vi "Threshold Windows Host.vi"() -> ()   [LabVIEW 2010]
uses:
  <vilib>/userDefined/High Color/nirio_resource_hc.ctl
  <vilib>/rvi/interface/nirviOpenFPGA/nirviOpenFPGA.xnode
  Threshold FPGA.vi
  <vilib>/rvi/interface/nirviOpenFPGA/nirviOpenFPGA.ctl
  <vilib>/rvi/interface/nirviOpenFPGA/nirviopenstate.ctl
  <vilib>/picture/picture.llb/imagedata.ctl
  <vilib>/rvi/interface/common/nirviIntfCommonState.ctl
  <vilib>/rvi/interface/common/nirviIntfModes.ctl
  Program Files/National Instruments/LabVIEW 2010/resource/RVI/emulation/niLvFpgaEmulationMode.ctl
  <vilib>/eio/XNode/Errors/EIOXNodeErrorStruct.ctl
  <vilib>/eio/XNode/Errors/EIOXNodeInternalErrorTypes.ctl
  <vilib>/eio/XNode/Errors/EIOXNodeUserErrorTypes.ctl
  <vilib>/XNodeSupport/XNodeRect32.ctl
  <vilib>/XNodeSupport/XNodeInt.ctl
  <vilib>/XNodeSupport/XNodeTerms.ctl
  <vilib>/XNodeSupport/XNodeTerm.ctl
  <vilib>/XNodeSupport/XNodeString.ctl
  <vilib>/XNodeSupport/XNodeVariant.ctl
  <vilib>/XNodeSupport/XNodeBool.ctl
  <vilib>/rvi/interface/nirviReadWriteControl/nirviReadWriteControl.xnode
  <vilib>/rvi/interface/nirviCloseFPGA/nirviCloseFPGA.xnode
  <vilib>/rvi/interface/RandomDataEmulation/nirviRandomDataOpen.vi
  <vilib>/rvi/interface/RandomDataEmulation/nirviRandomDataClose.vi
  <vilib>/XNodeSupport/NI_XNodeSupport.lvlib
panel:
  in  "Threshold (Volts)":dbl
  out "AI0 (Volts)":dbl
  in  "Stop Host":bool
  out "Threshold Exceeded":bool
  in  "Monitoring Loop Period (ms)":u32
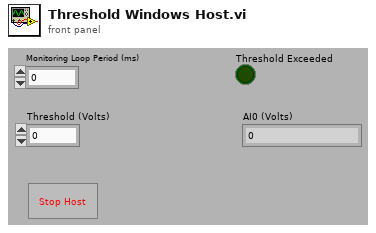
[diagram p1: front panel]
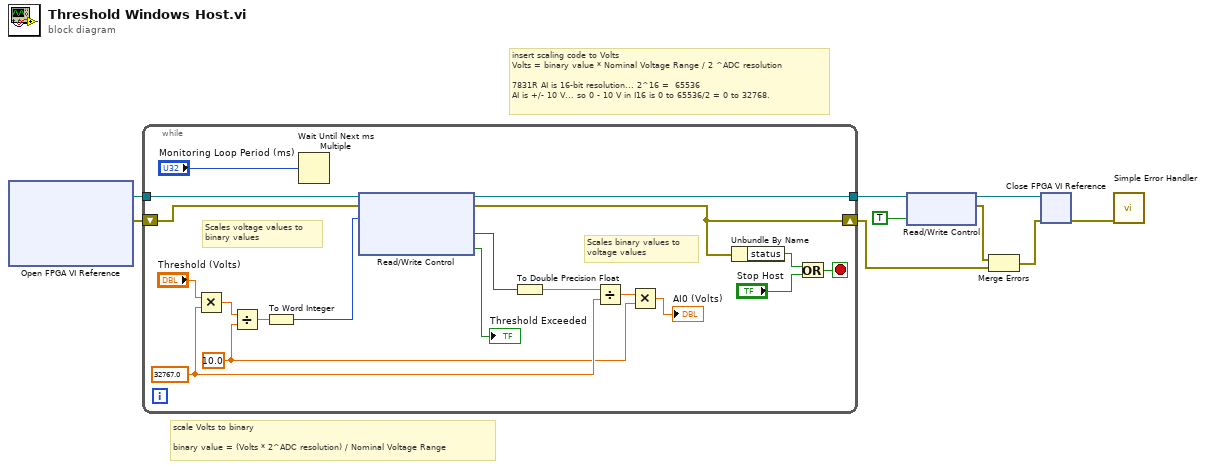
[diagram p0: block diagram]
diagram:
  # "scale Volts to binary\n\nbinary value = (Volts * 2^ADC resolution) / Nominal Voltage Range"
  # "insert scaling code to Volts\nVolts = binary value * Nominal Voltage Range / 2 ^ADC resolution\n\n7831R AI is 16-bit resolution... 2^16 =  65536\nAI is +/- 10 V... so 0 - 10 V in I16 is 0 to 65536/2 = 0 to 32768."
  n1 = xnode "Open FPGA VI Reference"() -> ("FPGA VI Reference Out"=w9:refnum<k20>, "error out"=w8:errorcluster)  [unwired: 2 in]
  n2 = while {
    tunnel: w9 -> [w28]
    tunnel: [w26] -> w5
    shift-right: [w24] -> w2
    shift-left: w8 -> [w25]
    stop <- w22 stop-if-true
    w12 = 10.0 ("y")
    w13 = 32767.0 ("y")
    # "Scales binary values to\nvoltage values"
    # "Scales voltage values to\nbinary values"
    n3 = Multiply(x="Threshold (Volts)", y=w13) -> (x*y=w20:dbl)
    n4 = Divide(x=w20, y=w12) -> (x/y=w19:dbl)
    n5 = To Word Integer(number=w19) -> (16bit integer=w15:i16)
    n6 = Wait Until Next ms Multiple(millisecond multiple="Monitoring Loop Period (ms)") -> ()  [unwired: 1 out]
    n7 = xnode "Read/Write Control"("FPGA VI Reference In"=w28, "error in"=w25, "Threshold (binary)"=w15) -> ("FPGA VI Reference Out"=w26:refnum<k20>, "error out"=w24:errorcluster, "AI0 (binary)"=w11:i16, "Threshold Exceeded"=→"Threshold Exceeded":bool)
    n8 = To Double Precision Float(number=w11) -> (double precision float=w10:dbl)
    n9 = Divide(x=w10, y=w13) -> (x/y=w18:dbl)
    n10 = Multiply(x=w18, y=w12) -> (x*y=→"AI0 (Volts)":dbl)
    n11 = Unbundle By Name "Unbundle By Name"(w24) -> ("status"=w23:bool)
    n12 = Or(x=w23, y="Stop Host") -> (x .or. y?=w22:bool)
  }
  n13 = xnode "Read/Write Control"("FPGA VI Reference In"=w5, "Stop FPGA"=TRUE) -> ("FPGA VI Reference Out"=w4:refnum<k20>, "error out"=w3:errorcluster)  [unwired: 1 in]
  n14 = Merge Errors(w3, w2) -> (w1:errorcluster)
  n15 = xnode "Close FPGA VI Reference"("FPGA VI Reference In"=w4, "error in"=w1) -> ("error out"=w7:errorcluster)
  n16 = call <vilib>:"Simple Error Handler.vi"("error in (no error)"=w7) -> ()  [unwired: 4 in, 5 out]
